vi "401_Update_audit_control.vi"(8 "error In":errorcluster, 11 "input cluster 2":T3) -> (0 "error Out":errorcluster)   [LabVIEW 2015]
uses:
  Utilities/TypeDefs/401_Audit_States.ctl
  <vilib>/addons/database/Connection.llb/Conn ObjectReference.ctl
  <vilib>/addons/database/NI_Database_API.lvlib
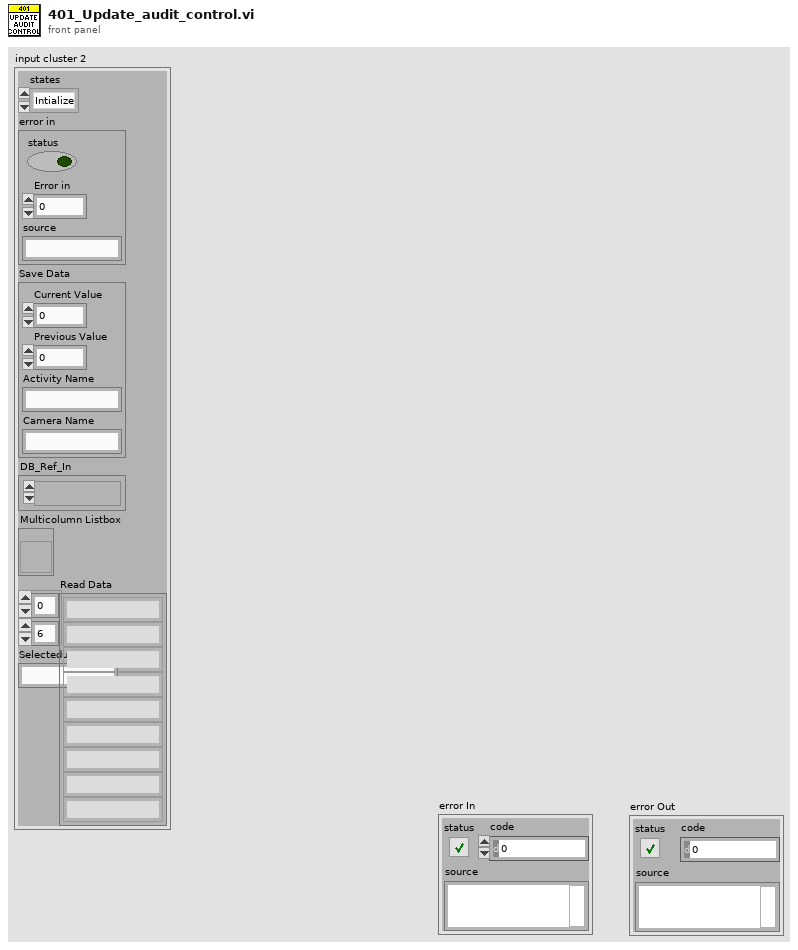
[diagram p1: front panel]
types:
  T1 = typedef "401_Audit_States.ctl" = enum16{"Intialize", "UpdateControls", "Save", "User Interface", "Finalize", "View User Data", "View Date time Data", "Add Audit Data", "Decending", "Ascending", "Export To Html", "UpdateFPCControls", "Quit"}
  T2 = typedef "NI_Database_API.lvlib/Conn ObjectReference.ctl" = refnum<k1>
  T3 = cluster{"states":T1, "error in":cluster{"status":bool, "Error in":i32, "source":string}, "Save Data":cluster{"Current Value":dbl, "Previous Value":dbl, "Activity Name":string, "Camera Name":string}, "DB_Ref_In":T2, "Multicolumn Listbox":refnum<vi>, "Read Data":string[][], "Selecteduser":string}
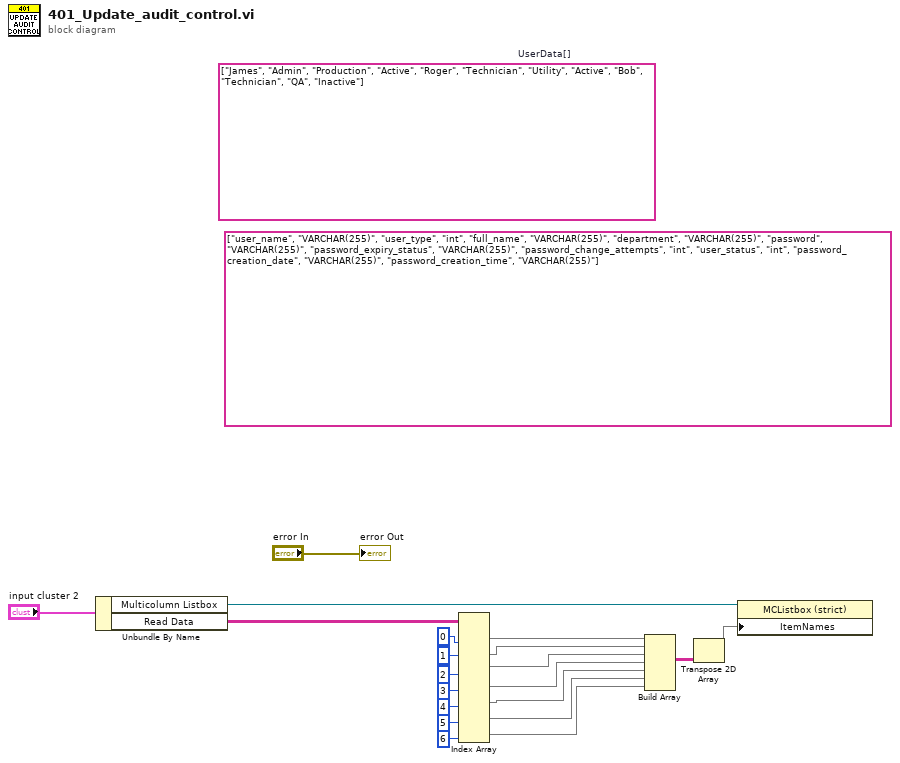
[diagram p0: block diagram]
diagram:
  (unwired) string[][] [["user_name", "VARCHAR(255)"], ["user_type", "int"], ["full_name", "VARCHAR(255)"], ["department", "VARCHAR(255)"], ["password", "VARCHAR(255)"], ["password_expiry_status", "VARCHAR(255)"], ["password_change_attempts", "int"], ["user_status", "int"], ["password_creation_date", "VARCHAR(255)"], ["password_creation_time", "VARCHAR(255)"]] ("ColoumnNames+DataType")
  (unwired) string[][] [["James", "Admin", "Production", "Active"], ["Roger", "Technician", "Utility", "Active"], ["Bob", "Technician", "QA", "Inactive"]]  # UserData[]
  n1 = Unbundle By Name("input cluster 2") -> ("Multicolumn Listbox"=w19:refnum<vi>, "Read Data"=w18:string[][])
  n2 = Index Array(array=w18, index (col) #1=0 ("disabled index (col)"), index (col) #2=1 ("index (col)"), index (col) #3=2 ("index (col)"), index (col) #4=3 ("index (col)"), index (col) #5=4 ("index (col)"), index (col) #6=5 ("index (col)"), index (col) #7=6 ("index (col)")) -> (element #1=w13:string[], element #2=w9:string[], element #3=w12:string[], element #4=w7:string[], element #5=w6:string[], element #6=w4:string[], element #7=w1:string[])  [unwired: 7 in]
  n3 = Build Array(w13, w9, w12, w7, w6, w4, w1) -> (w11:string[][])
  n4 = Transpose 2D Array(2D array=w11) -> (transposed array=w10:string[][])
  n5 = property class="MCListbox (strict)"(reference=w19, "ItemNames"=w10) -> ()  [unwired: 1 in, 2 out]
  "error Out" <- "error In"
